vi "ma_Formula Parser.vi"(2 "Reset":bool, 3 "Array":string[](array[string])=["-92.5", "-92.5+21.5*log2(f/4000)", "-34.5", "-34.5-48.0*log2(f/138000)"]) -> (0 "Variables":string[][](array[string]), 1 "Parsed Formula":cluster{"Table":i32[][], "Y Values":dbl[]}[](array[cluster]) {"Y Values" format="%0.2f"})   [LabVIEW 2020, in "NI_MAPro.lvlib"]
uses:
  NI_MAPro.lvlib
  NI_Gmath.lvlib
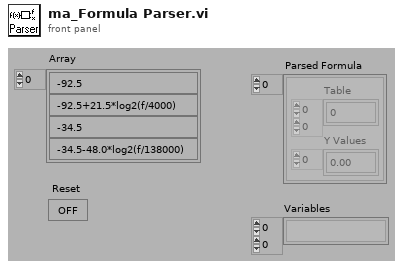
[diagram p1: front panel]
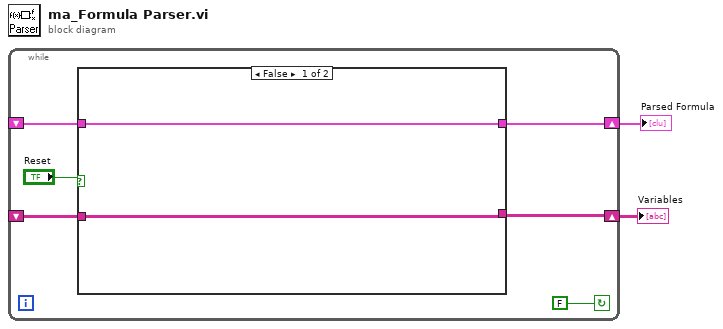
[diagram p0: block diagram]
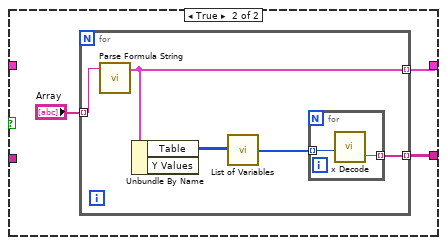
[diagram p2: hidden frame]
diagram:
  n1 = while {
    shift-left: _ -> [w7]
    shift-right: [w5] -> w1
    shift-left: _ -> [w8]
    shift-right: [w6] -> w2
    stop <- FALSE continue-if-true
    n2 = case shown="False" "Reset" {
      tunnel: [w9 w12] -> w5
      tunnel: [w10 w11] -> w6
      tunnel: w8 -> [w10 _]
      tunnel: w7 -> [w9 _]
      frame False {
      }
      frame True {
        n3 = for {
          tunnel: "Array" -> [w16] mode=indexing
          tunnel: [w15] -> w12 mode=indexing
          tunnel: [w14] -> w11 mode=indexing
          n4 = call "Parse Formula String.vi"("formula"=w16) -> ("Parsed Formula"=w14:cluster{"Table":i32[][], "Y Values":dbl[]})  [unwired: 1 in, 1 out]
          n5 = Unbundle By Name(w14) -> ("Table"=w17:i32[][])  [unwired: 1 out]
          n6 = call "List of Variables.vi"("Table"=w17) -> ("List of variables"=w18:i32[])
          n7 = for {
            tunnel: w18 -> [w20] mode=indexing
            tunnel: [w19] -> w15 mode=indexing
            n8 = call "x Decode.vi"("number"=w20) -> ("x string"=w19:string)  [unwired: 1 in, 1 out]
          }
        }
      }
    }
  }
  "Parsed Formula" <- w2
  "Variables" <- w1
